vi "Tilt_Reading.vi"(0 "Direction":enum16{"X", "Y", "Z"}(ring), 2 "SRV In":string) -> (1 "A/D Value":dbl, 4 "SRV Out":string="169.254.0.10")   [LabVIEW 2009]
panel:
  out "Reply":string
  # "This LabVIEW item is deprecated.\n\nIt is believed to be unused and will be removed in a future version of SRV."
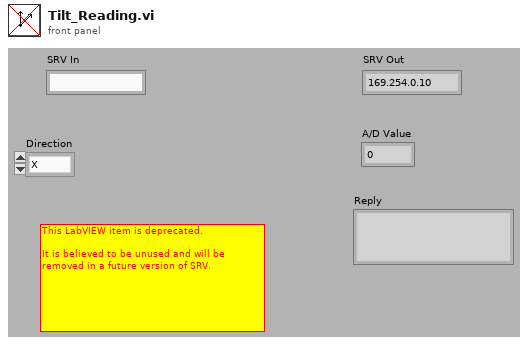
[diagram p1: front panel]
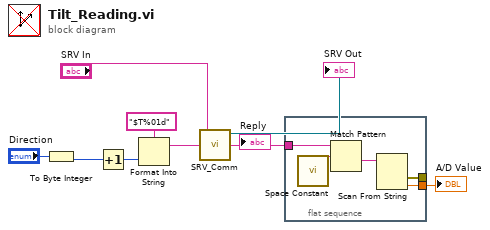
[diagram p0: block diagram]
diagram:
  n1 = To Byte Integer(number="Direction") -> (8bit integer=w1:i8)
  n2 = Increment(x=w1) -> (x+1=w2:i8)
  n3 = Format Into String(format string="$T%01d" ("Command Sent"), w2) -> (resulting string=w7:string)  [unwired: 2 in, 1 out]
  n4 = call "SRV_Comm.vi"("Command Sent"=w7, "SRV In"="SRV In") -> ("Reply"=w6:string, "SRV Out"=→"SRV Out":refnum<k5>)  [unwired: 1 in, 1 out]
  "Reply" <- w6
  n5 = flat-sequence {
    tunnel: w6 -> [w14]
    tunnel: [w13] -> w5
    tunnel: [w10] -> _
    frame #0 {
      n6 = call <vilib>:"Space Constant.vi"() -> ("String"=w12:string)
      n7 = Match Pattern(string=w14, regular expression=w12) -> (after substring=w11:string)  [unwired: 1 in, 3 out]
      n8 = Scan From String(input string=w11) -> (error out=w10:errorcluster, output 1=w13:dbl)  [unwired: 4 in, 2 out]
    }
  }
  "A/D Value" <- w5
